vi "CompletePerformance.vi"() -> ()   [LabVIEW 2015]
uses:
  ScaleAndLimitAI16Config.ctl
  AI16LimitsConfig.ctl
  AI16ScaleConfig.ctl
  <vilib>/Platform/TimedLoop/XDataNode/timing_clust.ctl
  <vilib>/Platform/TimedLoop/XDataNode/nitl_modes.ctl
  <vilib>/Platform/TimedLoop/XDataNode/wakeup.ctl
  SingleAIConfig.ctl
  <vilib>/rvi/Emulation/niFpgaGetClockAttributes.vi
  <vilib>/rvi/Emulation/niFpgaSctlEmulationGetInTimedLoop.vi
  <vilib>/rvi/Emulation/niFpgaEmulationReportErrorSimple.vi
  <vilib>/NI/PowerConversion/Utility/FPGA_Timers/TickTocks/Tick0.vi
  <vilib>/rvi/eio/common/nirviEmuTemplateMethod_errors.vi
  <vilib>/NI/PowerConversion/Utility/FPGA_Timers/TickTocks/Tock0.vi
  <vilib>/NI/PowerConversion/Utility/FPGA_Timers/TickTocks/Tick1.vi
  <vilib>/NI/PowerConversion/Utility/FPGA_Timers/TickTocks/Tick2.vi
  <vilib>/rvi/Emulation/niFpgaCriticalErrorInLSC.vi
  <vilib>/NI/PowerConversion/Utility/FPGA_Timers/TickTocks/Tock2.vi
  <vilib>/NI/PowerConversion/Utility/FPGA_Timers/TickTocks/Tock1.vi
  <vilib>/Platform/TimedLoop/XDataNode/XDataNode.xnode
  <vilib>/eio/EIONode/EIONode.xnode
  <vilib>/Platform/TimedLoop/XDataNode/XDNodeRunTimeDep.lvlib
  ScaleAndLimit.lvlib
  <vilib>/NI/PowerConversion/Utility/FPGA_Timers/Timers.lvlib
panel:
  out "MaxTimes":u32[](array[numeric])
  out "Times":u32[](array[numeric])
  in  "resetMaxTime":bool
  in  "InjectFault":bool
  out "loop time":u32
  out "AIFaulted":bool
  out "AIFaultHigh":u16 format="%.0b"
  out "AIFaultLow":u16 format="%.0x"
  in  "ClearFaults":bool
  out "ScaledAI":sgl[](array[numeric])
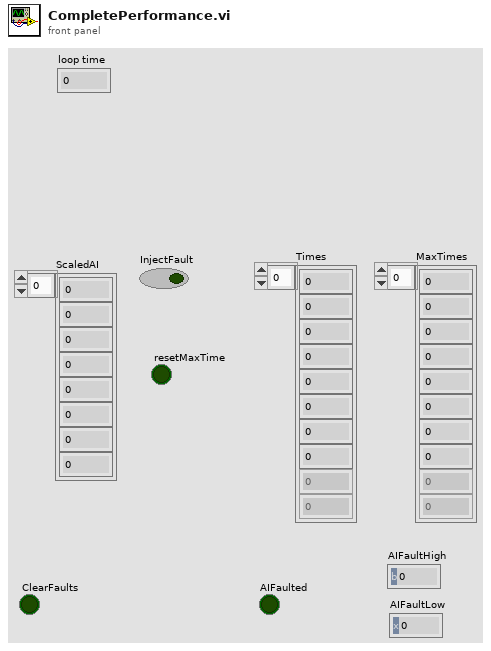
[diagram p1: front panel]
types:
  T1 = typedef "ScaleAndLimit.lvlib/ScaleAndLimitAI16Config.ctl" = cluster{"AI16Fault":T2, "AI16ScaleConfig":T3}
  T2 = typedef "ScaleAndLimit.lvlib/AI16LimitsConfig.ctl" = cluster{"LimitsEnabled":u16, "UnscaledHighLimit":i16[], "UnscaledLowLimit":i16[]}
  T3 = typedef "ScaleAndLimit.lvlib/AI16ScaleConfig.ctl" = cluster{"B":i16[], "M":sgl[]}
  T4 = typedef "ScaleAndLimit.lvlib/SingleAIConfig.ctl" = cluster{"LimitsEnable":bool, "UnscaledHighLimit":i16, "UnscaledLowLimit":i16, "B":i16, "M":sgl}
  T5 = typedef "Timers.lvlib/TimerRegisters.ctl" = cluster{"Tick0":refnum<k21>, "Tock0":refnum<k21>, "Tick1":refnum<k21>, "Tock1":refnum<k21>, "Tick2":refnum<k21>, "Tock2":refnum<k21>, "Tick3":refnum<k21>, "Tock3":refnum<k21>, "Tick4":refnum<k21>, "Tock4":refnum<k21>, "Tick5":refnum<k21>, "Tock5":refnum<k21>, "Tick6":refnum<k21>, "Tock6":refnum<k21>, "Tick7":refnum<k21>, "Tock7":refnum<k21>}
  T6 = typedef "XDNodeRunTimeDep.lvlib/timing_clust.ctl" = cluster{"Expected End [f-1]":u64, "Actual End [f-1]":u64, "Finished Late? [f-1]":bool, "Expected End [i-1]":u64, "Actual End [i-1]":u64, "Finished Late? [i-1]":bool, "Expected Start [i]":u64, "Actual Start [i]":u64, "Expected Start [f]":u64, "Actual Start [f]":u64, "Source Name":string, "Structure Name":string, "Period":i64, "Deadline":i64, "Offset":i64, "Start":i64, "Priority":i32, "Timeout":i32, "Mode":T7, "Wakeup Reason":T8, "Error":errorcluster, "Source Type":string, "Secondary Source Type":string, "Global End Time":u64, "Global Start Time":u64, "Frame Duration":u64, "Iteration Duration":u64, "Assigned CPU":i32, "I/O Scan Engine Mode":u32}
  T7 = typedef "XDNodeRunTimeDep.lvlib/nitl_modes.ctl" = enum32{"No Change", "Process missed periods, maintain original phase", "Discard missed periods, maintain original phase", "Process missed periods, ignore original phase", "Discard missed periods, ignore original phase"}
  T8 = typedef "XDNodeRunTimeDep.lvlib/wakeup.ctl" = enum32{"Normal", "Aborted", "Asynchronous wakeup", "Timing source error", "Timed loop error", "Timeout"}
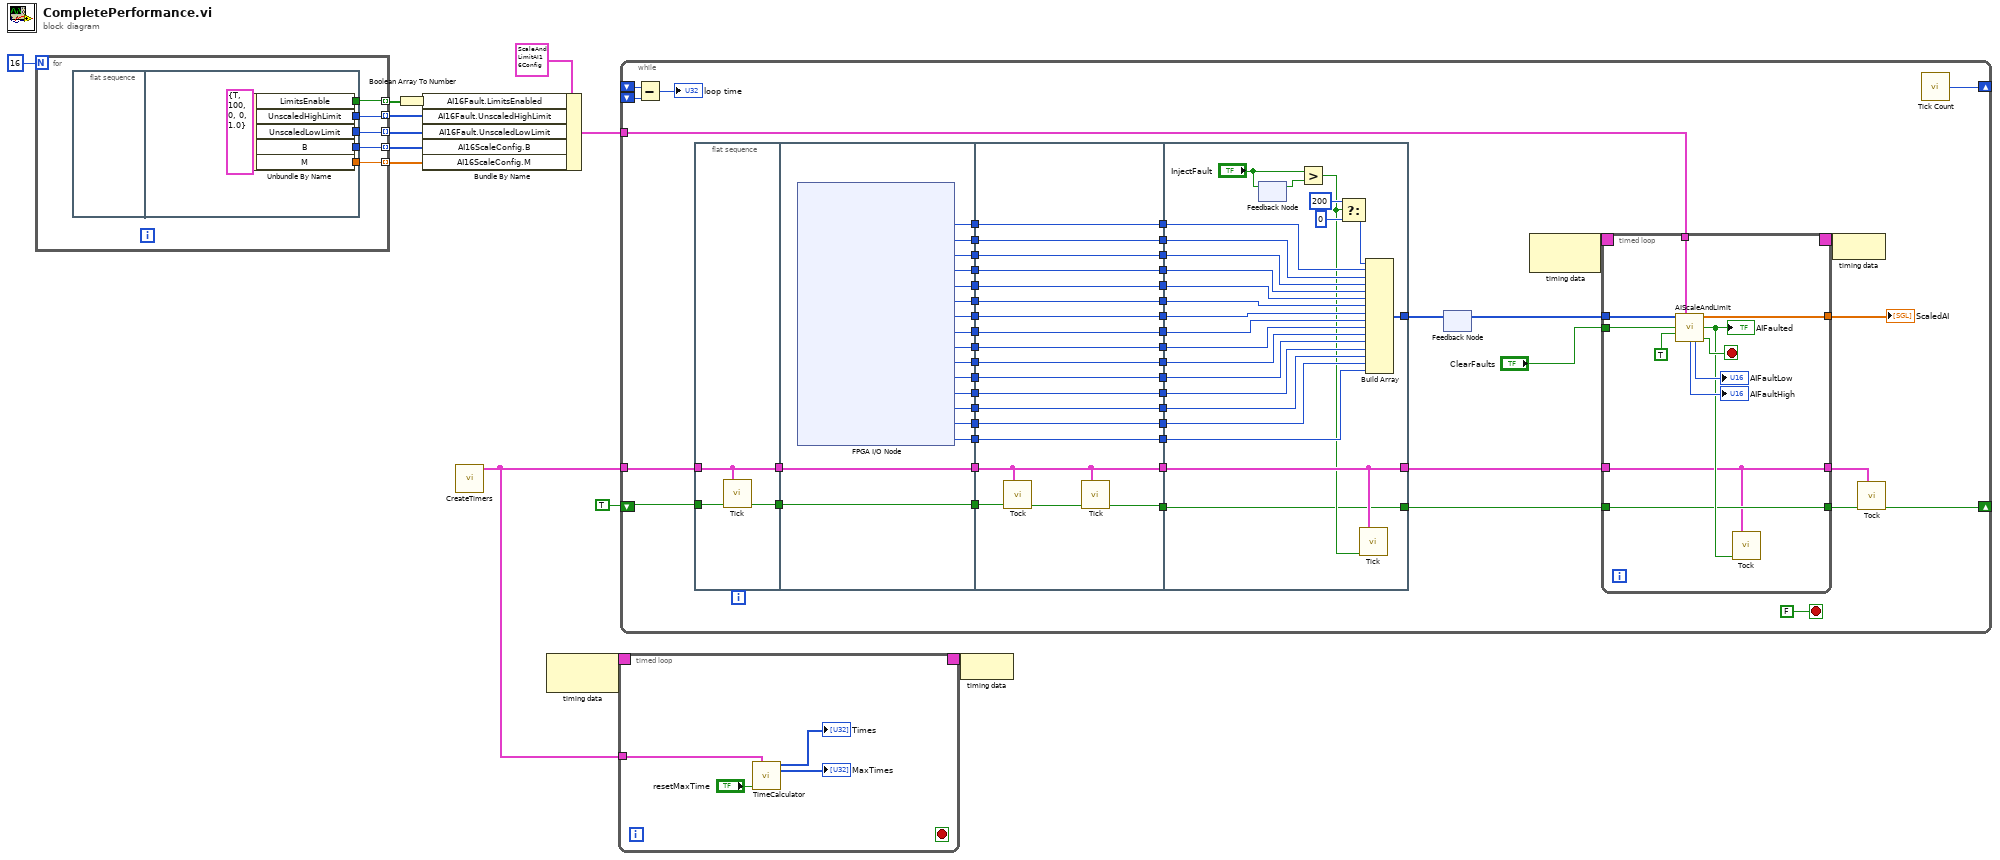
[diagram p0: block diagram]
diagram:
  n1 = for {
    N: 16 -> [_]
    tunnel: [w18] -> w11 mode=indexing
    tunnel: [w17] -> w8 mode=indexing
    tunnel: [w16] -> w7 mode=indexing
    tunnel: [w15] -> w6 mode=indexing
    tunnel: [w14] -> w5 mode=indexing
    n2 = flat-sequence {
      tunnel: [w23] -> w18
      tunnel: [w22] -> w17
      tunnel: [w21] -> w16
      tunnel: [w20] -> w15
      tunnel: [w19] -> w14
      frame #0 {
      }
      frame #1 {
        n3 = Unbundle By Name(T4 {"LimitsEnable"=TRUE, "UnscaledHighLimit"=100, "UnscaledLowLimit"=0, "B"=0, "M"=1.0} ("SingleAIConfig")) -> ("LimitsEnable"=w23:bool, "UnscaledHighLimit"=w22:i16, "UnscaledLowLimit"=w21:i16, "B"=w20:i16, "M"=w19:sgl)
      }
    }
  }
  n4 = Boolean Array To Number(Boolean array=w11) -> (number=w9:u16)
  n5 = Bundle By Name(cluster=T1 {"AI16Fault"={"LimitsEnabled"=0, "UnscaledHighLimit"=[0, 0, 0, 0, 0, 0, 0, 0, 0, 0, 0, 0, 0, 0, 0, 0], "UnscaledLowLimit"=[0, 0, 0, 0, 0, 0, 0, 0, 0, 0, 0, 0, 0, 0, 0, 0]}, "AI16ScaleConfig"={"B"=[0, 0, 0, 0, 0, 0, 0, 0, 0, 0, 0, 0, 0, 0, 0, 0], "M"=[0.0, 0.0, 0.0, 0.0, 0.0, 0.0, 0.0, 0.0, 0.0, 0.0, 0.0, 0.0, 0.0, 0.0, 0.0, 0.0]}} ("AIConfig"), "AI16Fault.LimitsEnabled"=w9, "AI16Fault.UnscaledHighLimit"=w8, "AI16Fault.UnscaledLowLimit"=w7, "AI16ScaleConfig.B"=w6, "AI16ScaleConfig.M"=w5) -> (w13:T1)
  n6 = call <vilib>:"CreateTimers.vi"() -> ("TimerRegisters"=w1:T5)  [unwired: 15 in]
  n7 = node-c288() -> (w3:T6)  [unwired: 1 in]
  n8 = timed-loop {
    timing: w3 -> [_]
    timing-out: [_] -> w2
    tunnel: w1 -> [w28]
    stop <- _ stop-if-true
    n9 = call <vilib>:"TimeCalculator.vi"("TimerRegisters"=w28, "resetMaxTime"="resetMaxTime") -> ("Times"=→"Times":u32[], "MaxTimes"=→"MaxTimes":u32[])  [unwired: 12 in]
  }
  n10 = while {
    shift-right: [w84] -> _
    shift-left: _ -> [w83]
    shift-left: _ -> [w82]
    tunnel: w13 -> [w80]
    tunnel: w1 -> [w74]
    shift-right: [w31] -> _
    shift-left: TRUE -> [w73]
    stop <- FALSE stop-if-true
    n11 = Subtract(x=w83, y=w82) -> (x-y=→"loop time":u32)
    n12 = flat-sequence {
      tunnel: w74 -> [w87]
      tunnel: w73 -> [w88]
      tunnel: [w87] -> w56
      tunnel: [w86] -> w54
      tunnel: [w105] -> w72
      tunnel: [w104] -> w71
      tunnel: [w103] -> w70
      tunnel: [w102] -> w69
      tunnel: [w101] -> w68
      tunnel: [w100] -> w67
      tunnel: [w99] -> w66
      tunnel: [w98] -> w65
      tunnel: [w97] -> w64
      tunnel: [w96] -> w63
      tunnel: [w95] -> w62
      tunnel: [w94] -> w61
      tunnel: [w93] -> w60
      tunnel: [w92] -> w59
      tunnel: [w91] -> w58
      tunnel: [w90] -> w57
      tunnel: w56 -> [w90]
      tunnel: [w89] -> w55
      tunnel: w54 -> [w89]
      tunnel: w72 -> [w124]
      tunnel: w71 -> [w123]
      tunnel: w70 -> [w122]
      tunnel: w69 -> [w121]
      tunnel: w68 -> [w120]
      tunnel: w67 -> [w119]
      tunnel: w66 -> [w118]
      tunnel: w65 -> [w117]
      tunnel: w64 -> [w116]
      tunnel: w63 -> [w115]
      tunnel: w62 -> [w114]
      tunnel: w61 -> [w113]
      tunnel: w60 -> [w112]
      tunnel: w59 -> [w111]
      tunnel: w58 -> [w110]
      tunnel: w57 -> [w107]
      tunnel: w55 -> [w109]
      tunnel: [w124] -> w53
      tunnel: [w123] -> w52
      tunnel: [w122] -> w51
      tunnel: [w121] -> w50
      tunnel: [w120] -> w49
      tunnel: [w119] -> w48
      tunnel: [w118] -> w47
      tunnel: [w117] -> w46
      tunnel: [w116] -> w45
      tunnel: [w115] -> w44
      tunnel: [w114] -> w43
      tunnel: [w113] -> w42
      tunnel: [w112] -> w41
      tunnel: [w111] -> w40
      tunnel: [w110] -> w39
      tunnel: [w107] -> w37
      tunnel: [w106] -> w35
      tunnel: w53 -> [w128]
      tunnel: w52 -> [w144]
      tunnel: w51 -> [w143]
      tunnel: w50 -> [w142]
      tunnel: w49 -> [w141]
      tunnel: w48 -> [w140]
      tunnel: w47 -> [w139]
      tunnel: w46 -> [w138]
      tunnel: w45 -> [w137]
      tunnel: w44 -> [w136]
      tunnel: w43 -> [w135]
      tunnel: w42 -> [w134]
      tunnel: w41 -> [w133]
      tunnel: w40 -> [w132]
      tunnel: w39 -> [w131]
      tunnel: [w130] -> w38
      tunnel: w37 -> [w127]
      tunnel: [w127] -> w36
      tunnel: w35 -> [w125]
      tunnel: [w125] -> w34
      frame #0 {
        n13 = call-poly <vilib>:"Tick.vi"("TimerRegisters"=w87, "valid input"=w88) -> ("valid output"=w86:bool)  [unwired: 13 in]
      }
      frame #1 {
        n14 = xnode "FPGA I/O Node"() -> ("RMC/Simultaneous/AI1"=w105:i16, "RMC/Simultaneous/AI2"=w104:i16, "RMC/Simultaneous/AI3"=w103:i16, "RMC/Simultaneous/AI4"=w102:i16, "RMC/Simultaneous/AI5"=w101:i16, "RMC/Simultaneous/AI6"=w100:i16, "RMC/Simultaneous/AI7"=w99:i16, "RMC/Simultaneous/AI8"=w98:i16, "RMC/Simultaneous/AI9"=w97:i16, "RMC/Simultaneous/AI10"=w96:i16, "RMC/Simultaneous/AI11"=w95:i16, "RMC/Simultaneous/AI12"=w94:i16, "RMC/Simultaneous/AI13"=w93:i16, "RMC/Simultaneous/AI14"=w92:i16, "RMC/Simultaneous/AI15"=w91:i16)  [unwired: 16 in, 17 out]
      }
      frame #2 {
        n15 = call-poly <vilib>:"Tock.vi"("TimerRegisters"=w107, "valid input"=w109) -> ("valid output"=w108:bool)  [unwired: 13 in]
        n16 = call-poly <vilib>:"Tick.vi"("TimerRegisters"=w107, "valid input"=w108) -> ("valid output"=w106:bool)  [unwired: 13 in]
      }
      frame #3 {
        n17 = feedback #1() -> (w145:bool)  [unwired: 1 in]
        n18 = feedback-in #1("InjectFault") -> ()
        n19 = Greater?(x="InjectFault", y=w145) -> (0:w126:bool)
        n20 = Select(t=i16 200, s=w126, f=i16 0 ("element")) -> (s? t:f=w129:i16)
        n21 = call-poly <vilib>:"Tick.vi"("TimerRegisters"=w127, "valid input"=w126) -> ()  [unwired: 13 in, 1 out]
        n22 = Build Array(w129, w128, w144, w143, w142, w141, w140, w139, w138, w137, w136, w135, w134, w133, w132, w131) -> (w130:i16[])
      }
    }
    n23 = feedback-in #2(w38) -> ()
    n24 = feedback #2() -> (w75:i16[])  [unwired: 1 in]
    n25 = node-c288() -> (w79:T6)  [unwired: 1 in]
    n26 = timed-loop {
      timing: w79 -> [_]
      timing-out: [_] -> w78
      tunnel: w75 -> [w149]
      tunnel: w80 -> [w153]
      tunnel: "ClearFaults" -> [w159]
      tunnel: [w157] -> w77
      tunnel: w36 -> [w150]
      tunnel: w34 -> [w151]
      tunnel: [w151] -> w33
      tunnel: [w150] -> w32
      stop <- w156 stop-if-true
      n27 = call "AIScaleAndLimit.vi"("UnscaledAI"=w149, "RawAIConfig"=w153, "ClearFaults"=w159, "input valid"=TRUE) -> ("ScaledAI"=w157:sgl[], "AIFaulted"=w152:bool, "AIFaultHigh"=→"AIFaultHigh":u16, "AIFaultLow"=→"AIFaultLow":u16, "output valid"=w156:bool)  [unwired: 6 in, 1 out]
      "AIFaulted" <- w152
      n28 = call-poly <vilib>:"Tock.vi"("TimerRegisters"=w150, "valid input"=w152) -> ()  [unwired: 13 in, 1 out]
    }
    "ScaledAI" <- w77
    n29 = node-c288(w78) -> ()
    n30 = call-poly <vilib>:"Tock.vi"("TimerRegisters"=w32, "valid input"=w33) -> ("valid output"=w31:bool)  [unwired: 13 in]
    n31 = call "Tick Count"() -> ("Tick Count(Ticks)"=w84:u32)
  }
  n32 = node-c288(w2) -> ()
